vi "rs3 get failed args.vi"(8 "error in (no error)":errorcluster, 11 "error in":u64) -> (0 "error out":errorcluster, 2 "error out":u64, 3 "Failed args":string)   [LabVIEW 2017, in "libRealSense3.lvlib"]
doc: "const char * rs_get_failed_args (const rs_error * error);"
uses:
  <vilib>/addons/RealSense/libRealSense3.lvlib
  <vilib>/addons/RealSense/realsense-d.dll
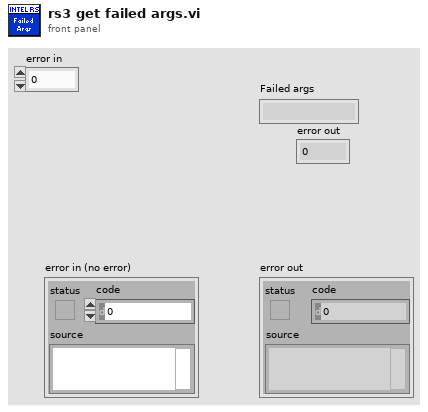
[diagram p1: front panel]
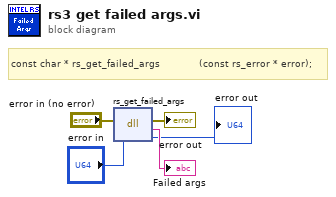
[diagram p0: block diagram]
diagram:
  # "const char * rs_get_failed_args             (const rs_error * error);"
  n1 = dll-call lib="C:/Program Files (x86)/National Instruments/LabVIEW 2017/vi.lib/addons/RealSense/realsense-d.dll" fn="rs_get_failed_args"(error in="error in (no error)", "error"="error in") -> (error out=→"error out":errorcluster, "return type"=→"Failed args":string, "error"=→"error out":u64)  [unwired: 2 in, 1 out]
